vi "Temp from Voltage Calculator.vi"(7 "error in (no error)":errorcluster, 10 "Graph Data 3":waveform(dbl)[](array[waveform])) -> (0 "error out":errorcluster, 3 "Graph Data 2":waveform(dbl)[](array[waveform]))   [LabVIEW 2023, in "Acquisition.lvlib"]
uses:
  Acquisition.lvlib
  <vilib>/express/express shared/ex_Modify Signal Name.vi
  <vilib>/express/express arith-compare/Formula/XNode/ExpressFormulaBlockNode.xnode
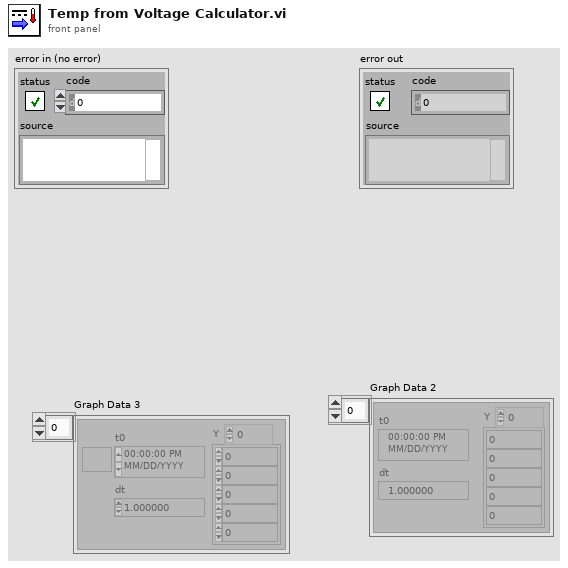
[diagram p1: front panel]
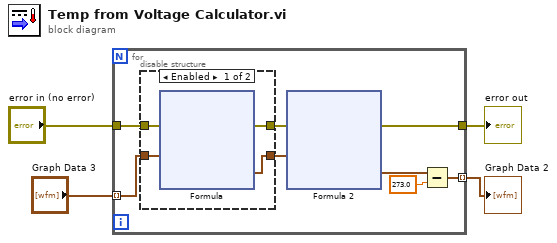
[diagram p0: block diagram]
diagram:
  n1 = for {
    tunnel: "Graph Data 3" -> [w8] mode=indexing
    tunnel: [w7] -> w3 mode=indexing
    tunnel: "error in (no error)" -> [w6]
    tunnel: [w5] -> w1
    n2 = disable-structure shown="Enabled" {
      disable-tunnel: [w16 w31] -> w10
      disable-tunnel: [w15 w32] -> w9
      disable-tunnel: w8 -> [w14 w31]
      disable-tunnel: w6 -> [w13 w32]
      frame Enabled {
        n3 = xnode "Formula"("v"=w14, "error in (no error)"=w13) -> ("Result"=w16:waveform(dbl), "error out"=w15:errorcluster)
      }
      frame Disabled {
      }
    }
    n4 = xnode "Formula 2"("R"=w10, "error in (no error)"=w9) -> ("Result"=w11:waveform(dbl), "error out"=w5:errorcluster)
    n5 = Subtract(x=w11, y=273.0) -> (x-y=w7:waveform(dbl))
  }
  "Graph Data 2" <- w3
  "error out" <- w1
